vi "测量主程序.vi"() -> ()   [LabVIEW 2018]
uses:
  Instr/_visa.llb/VISA Configure Serial Port (Instr).vi
panel:
  in  "Filename":string="6482_IV"
  in  "第N次测试":dbl
  out "错误输出":errorcluster
  in  "Completion Task":u16(ring) caption="完成任务" items=["保持Excel打开", "关闭电子表格"]
  out "error out":errorcluster caption="错误输出"
  in  "error in (no error)":errorcluster caption="错误输入（无错误）"
  in  "VISA资源名称":refnum<visa-resource-name>="COM15"
  in  "测量时间间隔(ms)":u32=1000
  in  "Vmax/Vc(V)":dbl=30.0
  in  "Vim(V)":dbl
  in  "间隔(V)":dbl=2.0
  out "电流大小":string="0.000000"
  out "Waveform Chart":dbl(graph)
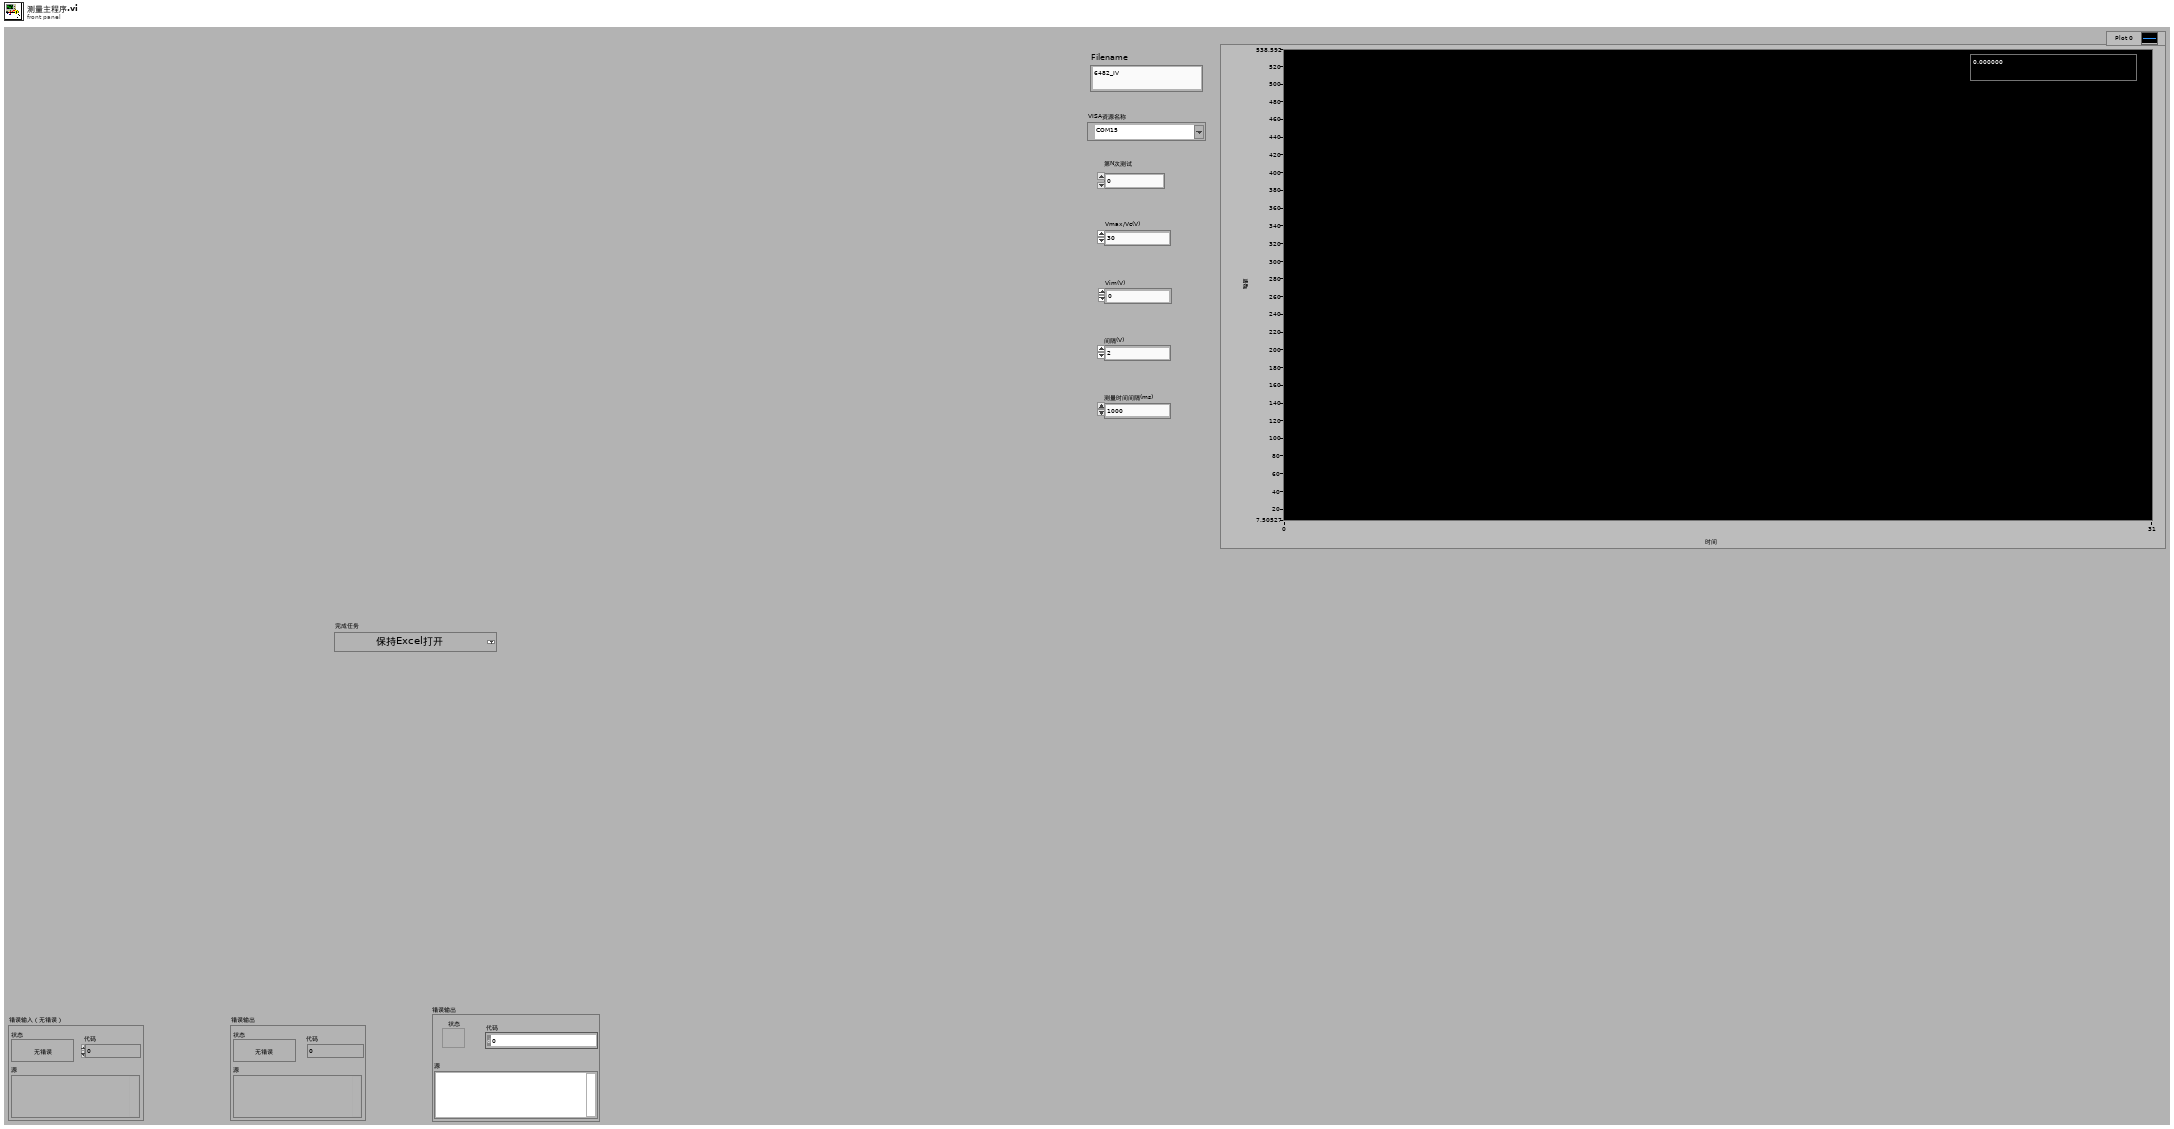
[diagram p1: front panel]
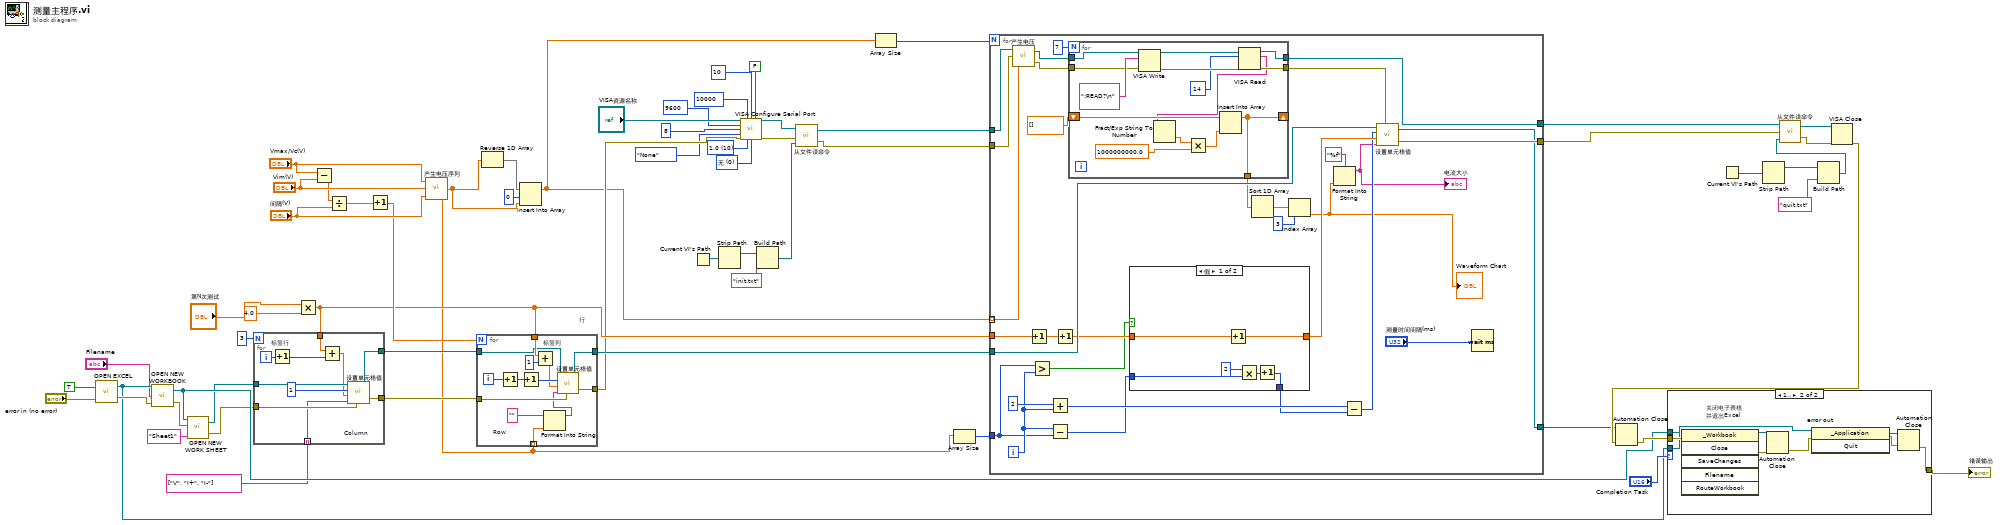
[diagram p0: block diagram]
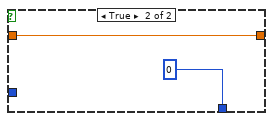
[diagram p2: hidden frame]
diagram:
  w4 = u16 0 items=["无", "XON/XOFF", "RTS/CTS", "XON/XOFF & RTS/CTS", "DTR/DSR", "XON/XOFF & DTR/DSR"] ("flow control (0:none)")
  w5 = u16 10 items=["1.0"=10, "1.5"=15, "2.0"=20] ("stop bits (10: 1 bit)")
  # "行"
  n1 = call "OPEN EXCEL.vi"("错误输入（无错误）"="error in (no error)", "Visible"=TRUE) -> ("错误输出"=w41:errorcluster, "引用输出"=w40:refnum<k7>)  [unwired: 1 in]
  n2 = call "OPEN NEW WORKBOOK.vi"("错误输入（无错误）"=w41, "Filename"="Filename", "Excel._Application"=w40) -> ("错误输出"=w37:errorcluster, "Excel._Application 2"=w38:refnum<k7>)
  n3 = call "OPEN NEW WORK SHEET.vi"("Sheet?"="Sheet1", "错误输入（无错误）"=w37, "Excel._Workbook"=w38) -> ("错误输出"=w35:errorcluster, "Excel._Worksheet"=w36:refnum<k7>)  [unwired: 1 in]
  n4 = Multiply(x="第N次测试", y=4.0) -> (x*y=w23:dbl)
  n5 = for {
    N: 3 -> [_]
    tunnel: w35 -> [w67]
    tunnel: [w70] -> w47
    tunnel: [w69] -> w46
    tunnel: string[] ["V", "I+", "I-"] -> [w65] mode=indexing
    tunnel: w23 -> [w68]
    tunnel: w36 -> [w66]
    i -> [w71]
    w64 = 1  # Column
    # "标签行"
    n6 = Increment(x=w71) -> (x+1=w62:i32)
    n7 = Add(x=w68, y=w62) -> (x+y=w63:dbl)
    n8 = call "设置单元格值.vi"("Excel._Worksheet 2"=w66, "Row"=w64, "Col"=w63, "Value"=w65, "error in (no error)"=w67) -> ("Excel._Worksheet"=w69:refnum<k7>, "error out"=w70:errorcluster)
  }
  n9 = Subtract(x="Vmax/Vc(V)", y="Vim(V)") -> (x-y=w28:dbl)
  n10 = Divide(x=w28, y="间隔(V)") -> (x/y=w26:dbl)
  n11 = Increment(x=w26) -> (x+1=w25:dbl)
  n12 = call "产生电压序列.vi"("Delt"="间隔(V)", "Min"="Vim(V)", "Max"="Vmax/Vc(V)") -> ("Array"=w1:dbl[])
  n13 = for {
    N: w25 -> [_]
    tunnel: w46 -> [w80]
    tunnel: w47 -> [w79]
    tunnel: [w84] -> w14
    tunnel: [w83] -> w24
    tunnel: w23 -> [w81]
    tunnel: w1 -> [w73] mode=indexing
    i -> [w76]
    w82 = 1  # Row
    # "标签列"
    n14 = Increment(x=w76) -> (x+1=w75:i32)
    n15 = Increment(x=w75) -> (x+1=w78:i32)
    n16 = Add(x=w81, y=w82) -> (x+y=w77:dbl)
    n17 = Format Into String(initial string="" ("初始字符串"), w73) -> (resulting string=w74:string)  [unwired: 2 in, 1 out]
    n18 = call "设置单元格值.vi"("Excel._Worksheet 2"=w80, "Row"=w78, "Col"=w77, "Value"=w74, "error in (no error)"=w79) -> ("Excel._Worksheet"=w83:refnum<k7>, "error out"=w84:errorcluster)
  }
  n19 = Reverse 1D Array(array=w1) -> (reversed array=w16:dbl[])
  n20 = Insert Into Array(array=w16, index=0 ("索引"), new element=w1) -> (w2:dbl[])
  n21 = Current VI's Path() -> (path=w60:path)
  n22 = Strip Path(path=w60) -> (stripped path=w59:path)  [unwired: 1 out]
  n23 = call-poly "VISA Configure Serial Port"("VISA resource name"="VISA资源名称", "timeout (10sec)"=u32 10000, "termination char\n(0xA = '\\n' = LF)"=u8 10 ("termination char\n(0xA = '\\n' = LF)"), "Enable Termination\nChar (T)"=FALSE ("Enable Termination\nChar (T)"), "baud rate (9600)"=u32 9600, "data bits (8)"=u16 8, "parity (0:none)"=enum16{"None", "Odd", "Even", "Mark", "Space"}."None", "error in (no error)"=w14, "stop bits (10: 1 bit)"=w5, "flow control (0:none)"=w4) -> ("VISA resource name out"=w13:refnum<visa-resource-name>, "error out"=w61:errorcluster)  [unwired: 4 in]
  n24 = Build Path(base path=w59, name or relative path="init.txt") -> (appended path=w57:path)
  n25 = call "从文件读命令.vi"("Path"=w57, "VISA error in"=w61, "VISA resource name"=w13) -> ("VISA error out"=w18:errorcluster, "VISA resource name out"=w19:refnum<visa-resource-name>)
  n26 = Array Size(array=w2) -> (size(s)=w20:i32)
  n27 = Array Size(array=w1) -> (size(s)=w15:i32)
  n28 = for {
    N: w20 -> [_]
    tunnel: w2 -> [w98] mode=indexing
    tunnel: w19 -> [w96]
    tunnel: w18 -> [w95]
    tunnel: [w92] -> w50
    tunnel: [w114] -> w49
    tunnel: w24 -> [w113]
    tunnel: w23 -> [w110]
    tunnel: [w112] -> w21
    tunnel: w15 -> [w105]
    i -> [w106]
    n29 = call "产生电压.vi"("volt"=w98, "VISA error in"=w95, "VISA resource name"=w96) -> ("VISA error out"=w93:errorcluster, "VISA resource name out"=w97:refnum<visa-resource-name>)
    n30 = Increment(x=w110) -> (x+1=w111:dbl)
    n31 = Greater?(x=w105, y=w106) -> (0:w107:bool)
    n32 = Add(x=2, y=w106) -> (x+y=w104:i32)
    n33 = Subtract(x=w106, y=w105) -> (x-y=w102:i32)
    n34 = Increment(x=w111) -> (x+1=w109:dbl)
    n35 = for {
      N: 7 -> [_]
      tunnel: w97 -> [w128]
      tunnel: [w123] -> w92
      tunnel: w93 -> [w124]
      tunnel: [w122] -> w91
      shift-right: [w117] -> _
      shift-left: dbl[] [] -> [w118]
      tunnel: [w117] -> w89
      n36 = VISA Write(VISA resource name=w128, write buffer=":READ?\n" ("写入缓冲区"), error in (no error)=w124) -> (VISA resource name out=w127:refnum<visa-resource-name>, error out=w126:errorcluster)  [unwired: 1 out]
      n37 = VISA Read(VISA resource name=w127, byte count=u32 14 ("字节总数"), error in (no error)=w126) -> (VISA resource name out=w123:refnum<visa-resource-name>, read buffer=w116:string, error out=w122:errorcluster)  [unwired: 1 out]
      n38 = Fract/Exp String To Number(string=w116) -> (number=w121:dbl)  [unwired: 3 in, 1 out]
      n39 = Multiply(x=w121, y=1000000000.0) -> (x*y=w119:dbl)
      n40 = Insert Into Array(array=w118, new element=w119) -> (w117:dbl[])  [unwired: 1 in]
    }
    n41 = case shown="假" w107 {
      tunnel: w109 -> [w135 w137]
      tunnel: [w134 w137] -> w108
      tunnel: [w130 0] -> w103
      tunnel: w102 -> [w133 _]
      frame False {
        n42 = Increment(x=w135) -> (x+1=w134:dbl)
        n43 = Multiply(x=2, y=w133) -> (x*y=w131:i32)
        n44 = Increment(x=w131) -> (x+1=w130:i32)
      }
      frame True {
      }
    }
    n45 = Sort 1D Array(array=w89) -> (sorted array=w88:dbl[])
    n46 = Index Array(array=w88, index=3 ("索引")) -> (element=w86:dbl)
    "Waveform Chart" <- w86
    n47 = Format Into String(format string="%f" ("格式字符串"), w86) -> (resulting string=w100:string)  [unwired: 2 in, 1 out]
    "电流大小" <- w100
    n48 = Subtract(x=w104, y=w103) -> (x-y=w101:i32)
    n49 = call "设置单元格值.vi"("Excel._Worksheet 2"=w113, "Row"=w101, "Col"=w108, "Value"=w100, "error in (no error)"=w91) -> ("Excel._Worksheet"=w112:refnum<k7>, "error out"=w114:errorcluster)
    n50 = Wait (ms)(milliseconds to wait="测量时间间隔(ms)") -> ()  [unwired: 1 out]
  }
  n51 = Current VI's Path() -> (path=w54:path)
  n52 = Strip Path(path=w54) -> (stripped path=w55:path)  [unwired: 1 out]
  n53 = Build Path(base path=w55, name or relative path="quit.txt") -> (appended path=w51:path)
  n54 = call "从文件读命令.vi"("Path"=w51, "VISA error in"=w49, "VISA resource name"=w50) -> ("VISA error out"=w52:errorcluster, "VISA resource name out"=w53:refnum<visa-resource-name>)
  n55 = VISA Close(VISA resource name=w53, error in (no error)=w52) -> (error out=w22:errorcluster)
  n56 = Automation Close(3:w22, 5:w21) -> (0:w45:errorcluster)
  n57 = case shown="1.." "Completion Task" {
    tunnel: w45 -> [w138 w142]
    tunnel: w40 -> [_ w141]
    tunnel: w38 -> [_ w140]
    tunnel: [w138 w139] -> w39
    frame ..0 {
    }
    frame 1.. {
      # "关闭电子表格\n并退出Excel"
      n58 = invoke class="_Workbook" method="Close"(reference=w140, error in=w142) -> (reference out=w147:refnum<k7>, error out=w146:errorcluster)  [unwired: 4 in, 4 out]
      n59 = Automation Close(3:w146, 5:w147) -> (0:w145:errorcluster)
      n60 = invoke class="_Application" method="Quit"(reference=w141, error in=w145) -> (reference out=w143:refnum<k7>, error out=w144:errorcluster)  [unwired: 1 in, 1 out]
      n61 = Automation Close(3:w144, 5:w143) -> (0:w139:errorcluster)
    }
  }
  "错误输出" <- w39
